vi "Controller Exit Cleanup.vi"(8 "error in (no error)":errorcluster, 11 "Actor_Controller_Template in":refnum<class "Actor_Controller_Template.lvclass">) -> (0 "error out":errorcluster, 3 "Actor_Controller_Template out":refnum<class "Actor_Controller_Template.lvclass">)   [LabVIEW 2020, in "Actor_Controller_Template.lvlib" / "Actor_Controller_Template.lvclass"]
uses:
  Actor_Controller_Template.lvclass
  Actor_UI_Template/UI Action Enum.ctl
  Actor_Controller_Template.lvclass/Actor_Controller_Template.ctl
  Actor_UI_Template/Actor_UI_Template Messages/Do UI Action Msg/Do UI Action Msg.lvclass/Do UI Action Msg.ctl
  <vilib>/ActorFramework/Message Enqueuer/Message Enqueuer.lvclass/Message Enqueuer.ctl
  <vilib>/ActorFramework/Message Enqueuer/Enqueue.vi
  Actor_UI_Template/Actor_UI_Template Messages/Do UI Action Msg/Do UI Action Msg.lvclass
  C:/Program Files/National Instruments/LabVIEW 2020/vi.lib/ActorFramework/Message/Message.lvclass
  <vilib>/ActorFramework/Message Priority Queue/Priority Enqueue.vi
  Actor_UI_Template/Actor_UI_Template.lvlib
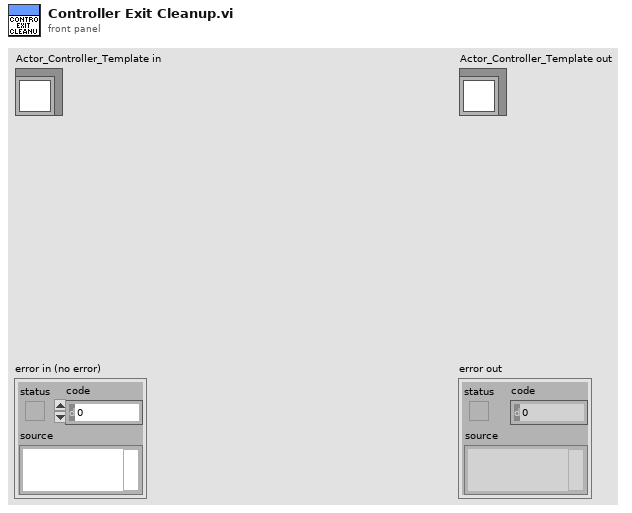
[diagram p1: front panel]
types:
  T1 = typedef "Actor_UI_Template.lvlib/UI Action Enum.ctl" = enum16{"Do UI Close"}
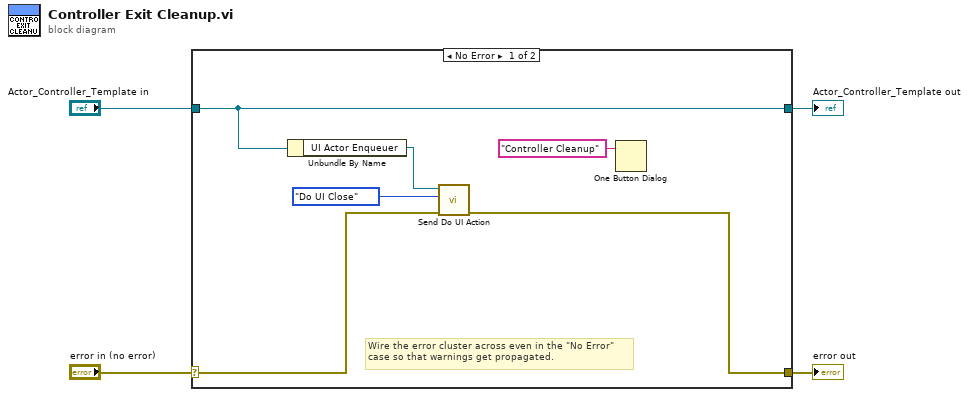
[diagram p0: block diagram]
diagram:
  n1 = case shown="No Error" "error in (no error)" {
    selector: "error in (no error)" -> [w7 w12]
    tunnel: [w6 w12] -> w3
    tunnel: [w10 w11] -> w1
    tunnel: "Actor_Controller_Template in" -> [w10 w11]
    frame No Error {
      # "Wire the error cluster across even in the \"No Error\"\ncase so that warnings get propagated."
      n2 = Unbundle By Name(w10) -> ("UI Actor Enqueuer"=w9:refnum<class "Message Enqueuer.lvclass">)
      n3 = call "Send Do UI Action.vi"("error in (no error)"=w7, "UI Action"=UI_Action_Enum."Do UI Close", "Message Enqueuer"=w9) -> ("error out"=w6:errorcluster)  [unwired: 7 in, 1 out]
      n4 = One Button Dialog(message="Controller Cleanup") -> ()  [unwired: 1 in, 1 out]
    }
    frame Error {
    }
  }
  "error out" <- w3
  "Actor_Controller_Template out" <- w1
